vi "Complete Elliptic Integral K.vi"(11 "k":dbl format="%.2f") -> (3 "K(k)":dbl format="%.2f")   [LabVIEW 2020, in "NI_Gmath.lvlib"]
doc: "Computes the Legendre elliptic integral of the first kind. You must manually select the polymorphic instance you want to use."
uses:
  <vilib>/gmath/NI_Gmath.lvlib
  <resource>/lvanlys.dll
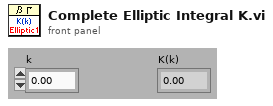
[diagram p1: front panel]
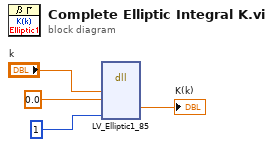
[diagram p0: block diagram]
diagram:
  n1 = dll-call lib="e:/builds/penguin/labview/branches/2020/dev/dist/resource/lvanlys.*" fn="LV_Elliptic1_85"("k"="k", "a"=0.0, "funcType"=1) -> ("Elliptic1(k, a)"=→"K(k)":dbl)  [unwired: 8 in, 2 out]
